vi "rp_merge_icon.vi"(6 "Variant in":variant, 7 "Shift Pressed?":bool, 8 "error in (no error)":errorcluster, 10 "QD Combo Box Ref":refnum<vi>, 11 "QD Launch VI Ref":refnum<vi>) -> (0 "error out":errorcluster, 4 "Variant out":variant)   [LabVIEW 2019]
doc: "Merge all icon layers to minimize space and avoid layer template collisions.\n\nCreated by: Ryan Pacini\n\nDefault Shortcut - [M]"
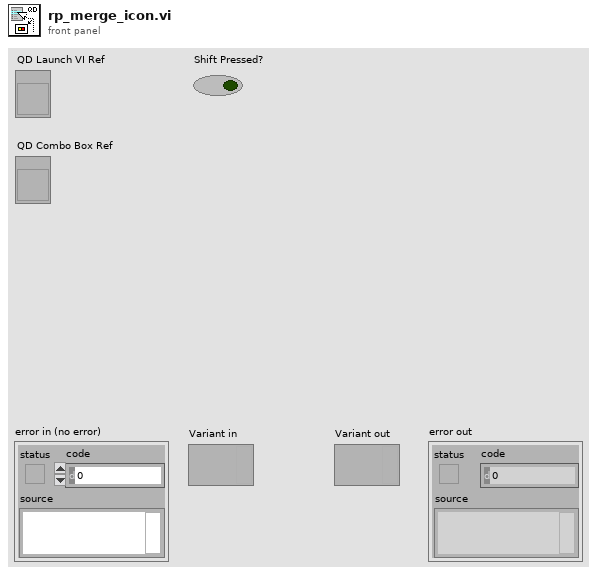
[diagram p1: front panel]
types:
  T1 = typedef "imagedata.ctl" = cluster{"image type":i32, "image depth":i32, "image":u8[], "mask":u8[], "colors":u32[], "Rectangle":cluster{"left":i16, "top":i16, "right":i16, "bottom":i16}}
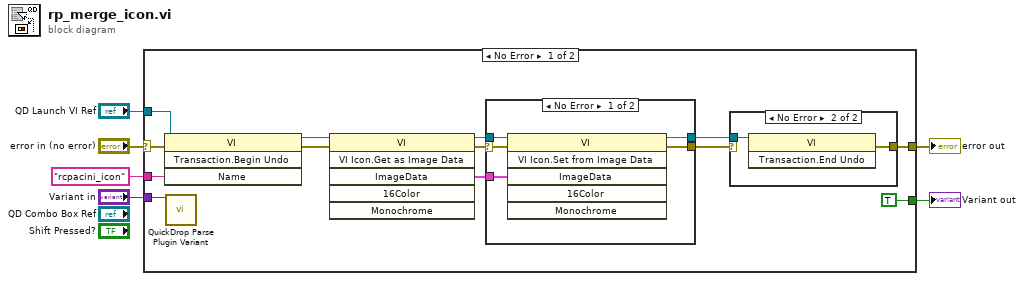
[diagram p0: block diagram]
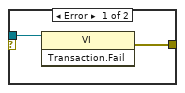
[diagram p3: hidden frame]
diagram:
  n1 = case shown="No Error" "error in (no error)" {
    selector: "error in (no error)" -> [w19 w31]
    tunnel: [w18 w31] -> w2
    tunnel: "QD Launch VI Ref" -> [w15 _]
    tunnel: "rcpacini_icon" ("Undo Name") -> [w17 _]
    tunnel: [TRUE _] -> w3
    tunnel: "Variant in" -> [w7 _]
    frame No Error {
      n2 = invoke class="VI" method="Transaction.Begin Undo"(reference=w15, error in=w19, "Name"=w17) -> (reference out=w10:refnum<vi>, error out=w11:errorcluster)  [unwired: 1 in, 2 out]
      n3 = call <vilib>:"QuickDrop Parse Plugin Variant.vi"("QDKS Variant in"=w7) -> ()  [unwired: 12 in, 3 out]
      n4 = invoke class="VI" method="VI Icon.Get as Image Data"(reference=w10, error in=w11) -> (reference out=w14:refnum<vi>, error out=w12:errorcluster, "ImageData"=w13:T1)  [unwired: 4 in, 3 out]
      n5 = case shown="No Error" w12 {
        selector: w12 -> [w22 w26]
        tunnel: w14 -> [w24 w25]
        tunnel: w13 -> [w23 _]
        tunnel: [w21 w26] -> w9
        tunnel: [w20 w25] -> w8
        frame No Error {
          n6 = invoke class="VI" method="VI Icon.Set from Image Data"(reference=w24, error in=w22, "ImageData"=w23) -> (reference out=w20:refnum<vi>, error out=w21:errorcluster)  [unwired: 3 in, 4 out]
        }
        frame Error {
        }
      }
      n7 = case shown="No Error" w9 {
        tunnel: w8 -> [w27 w29]
        tunnel: [w28 w30] -> w18
        frame Error {
          n8 = invoke class="VI" method="Transaction.Fail"(reference=w27) -> (error out=w28:errorcluster)  [unwired: 2 in, 2 out]
        }
        frame No Error {
          n9 = invoke class="VI" method="Transaction.End Undo"(reference=w29) -> (error out=w30:errorcluster)  [unwired: 2 in, 2 out]
        }
      }
    }
    frame Error {
    }
  }
  "error out" <- w2
  "Variant out" <- w3
